vi "Update position.vi"(8 "error in (no error)":errorcluster, 11 "StageSPIM in":refnum<class "StageSPIM.lvclass">) -> (0 "error out":errorcluster, 3 "StageSPIM out":refnum<class "StageSPIM.lvclass">)   [LabVIEW 2012, in "StageSPIM.lvclass"]
uses:
  StageSPIM.lvclass
  StageSPIM.lvclass/StageSPIM.ctl
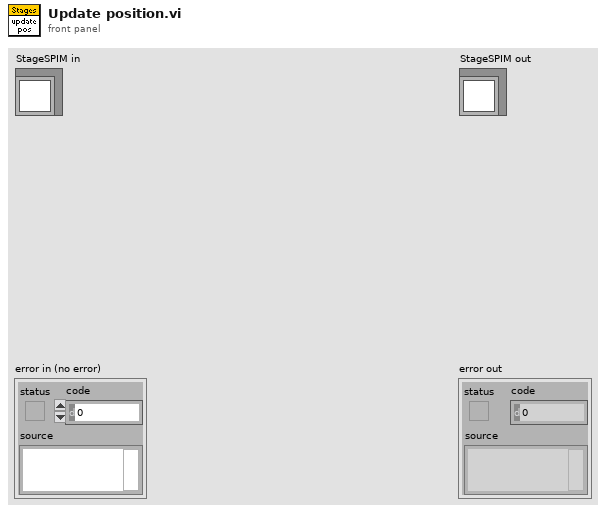
[diagram p1: front panel]
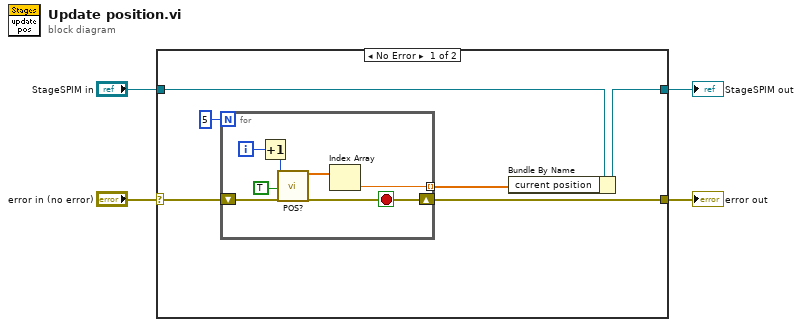
[diagram p0: block diagram]
diagram:
  n1 = case shown="No Error" "error in (no error)" {
    selector: "error in (no error)" -> [w9 w19]
    tunnel: [w8 w19] -> w3
    tunnel: [w5 w18] -> w1
    tunnel: "StageSPIM in" -> [w6 w18]
    frame No Error {
      n2 = for {
        N: 5 -> [_]
        shift-right: [w11] -> w8
        shift-left: w9 -> [w17]
        tunnel: [w12] -> w7 mode=indexing
        i -> [w16]
        stop <- w11 stop-if-true
        n3 = Increment(x=w16) -> (x+1=w15:i32)
        n4 = call "POS?.vi"("System no."=w15, "All axes?"=TRUE, "error in"=w17) -> ("Position"=w13:dbl[], "error out"=w11:errorcluster)  [unwired: 15 in]
        n5 = Index Array(array=w13) -> (element=w12:dbl)  [unwired: 1 in]
      }
      n6 = Bundle By Name(cluster=w6, "current position"=w7) -> (w5:refnum<class "StageSPIM.lvclass">)
    }
    frame Error {
    }
  }
  "error out" <- w3
  "StageSPIM out" <- w1
